vi "VM_Projeto.vi"() -> ()   [LabVIEW 2016]
uses:
  <vilib>/vision/Pattern Matching.llb/IMAQ Match Range Setting.ctl
  <vilib>/vision/Pattern Matching.llb/IMAQ Curve Parameters.ctl
  <vilib>/Analysis/_algsub.llb/Vector Norm Type.ctl
  <vilib>/Analysis/_algsub.llb/Real Vector Norm.vi
  <vilib>/vision/NI_Vision_Development_Module.lvlib
  <vilib>/Analysis/NI_AALPro.lvlib
panel:
  out "Array 5":i32[](array[numeric])
  out "reversed array":i32[](array[numeric])
  in  "stop":bool
  out "Array 4":T1[](array[typedef]) {"Contours"."Type" items=["No Selection", "Point", "Line", "Rectangle", "Oval", "Polygon", "Freehand Region", "Annulus", "Unused2", "Unused3", "Broken Line", "Freehand Line", "Rotated Rectangle"]}
  out "Array 3":cluster{"x":sgl, "y":sgl}[](array[cluster])
  out "Array 2":sgl[](array[numeric])
  out "Array":dbl[][](array[numeric])
  out "Number of Matches (filtered)":i32
  out "Number of Matches":i32
  in  "Number of Matches Requested":i32=40 min=1
  in  "Minimum Match Score":sgl=975.0 min=0 max=1000 format="%.2f"
  in  "Template":path=path "C:/Users/Alexandre/Documents/LabView Projects/Projeto/template.png"
  out "Image Out 2":T2(plugin-control)
  out "Image Out":T2(plugin-control)
  in  "Base":path=path "C:/Users/Alexandre/Documents/LabView Projects/Projeto/base.jpg"
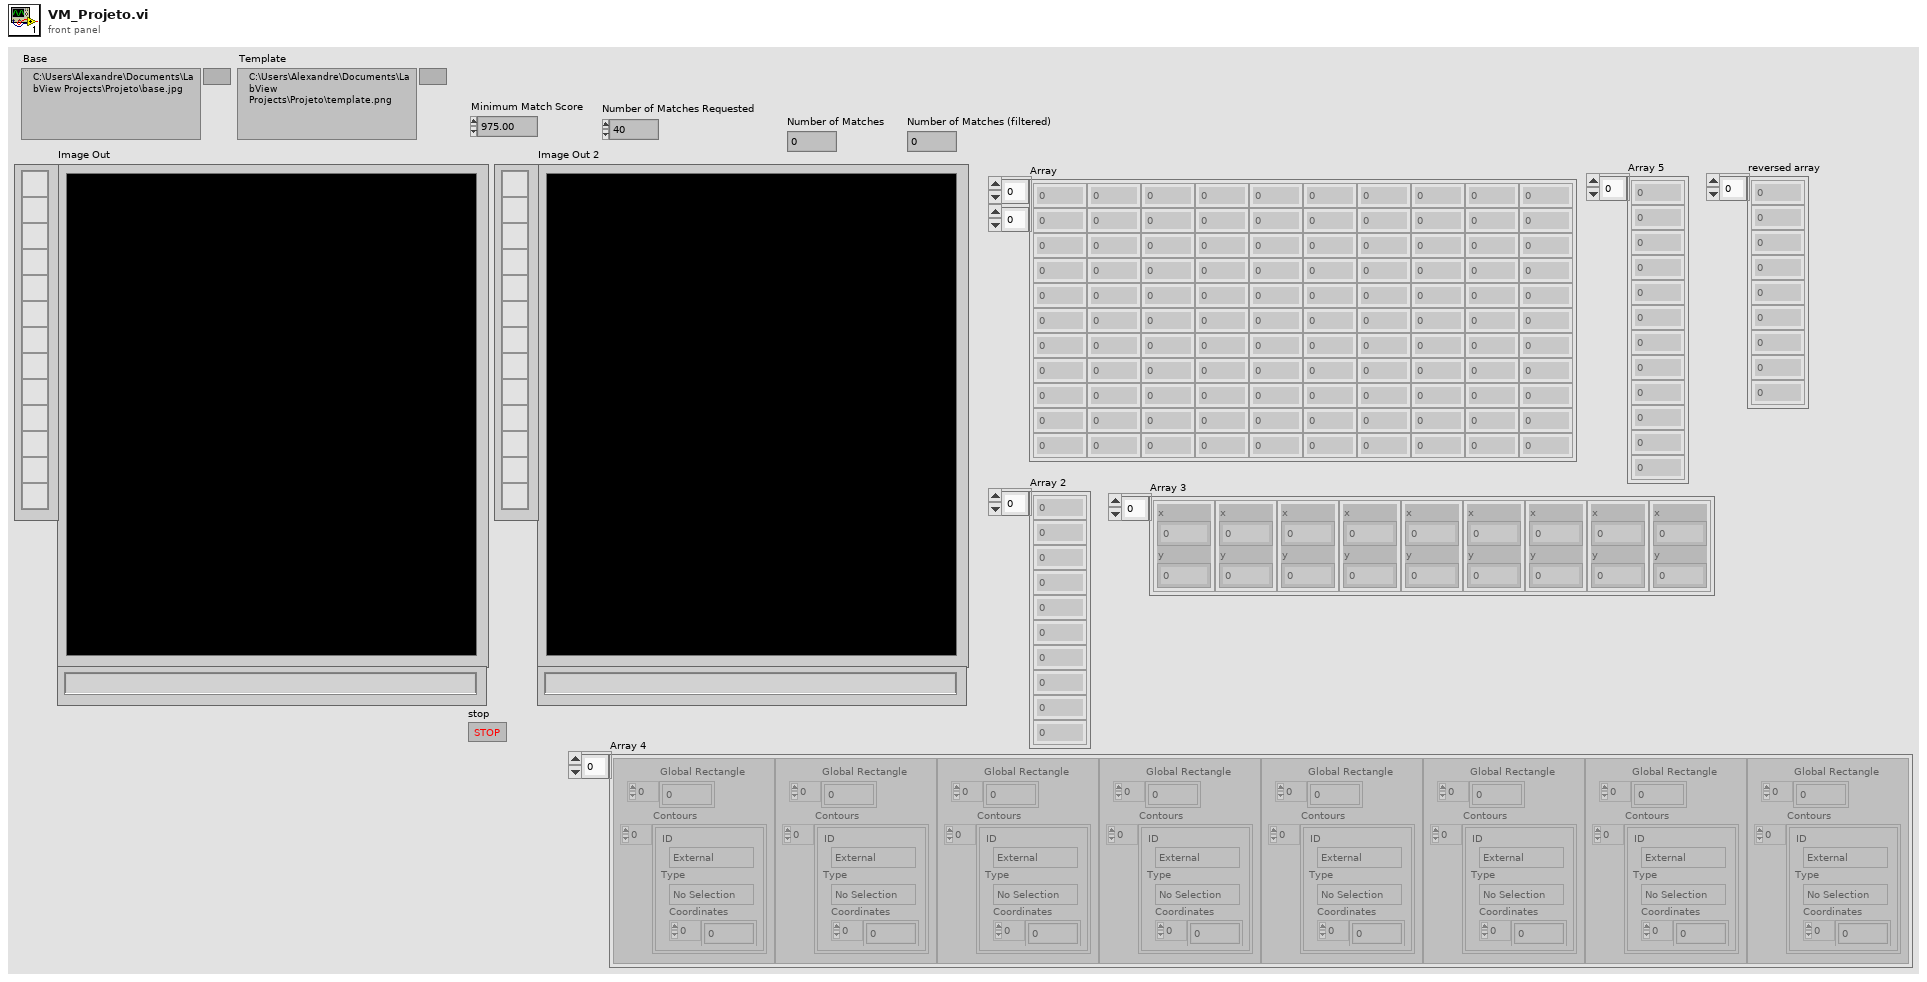
[diagram p1: front panel]
types:
  T1 = typedef "ROI Descriptor" = cluster{"Global Rectangle":i32[], "Contours":cluster{"ID":enum32{"External", "Internal"}, "Type":u32, "Coordinates":i32[]}[]}
  T2 = typedef "IMAQ Image.ctl" = refnum<image>
  T3 = typedef "IMAQ Curve Parameters.ctl" = cluster{"Extraction Mode":u32, "Edge Threshold":i32, "Edge Filter Size":u32, "Min Length":i32, "Row Search Step Size":i32, "Col Search Step Size":i32, "Max Endpoint Gap":i32, "Closed":bool, "Subpixel":bool}
  T4 = cluster{"Setup Data Item":u16, "Item Value":dbl}[]
  T5 = cluster{"Rotation":bool, "Scale":bool, "Occlusion":bool, "Reserved":bool, "Reserved":bool, "Reserved":bool}
  T6 = typedef "IMAQ Match Range Setting.ctl" = cluster{"Match Constraints":u32, "Min":dbl, "Max":dbl}
  T7 = typedef "IMAQ Rectangle" = cluster{"Left":i32, "Top":i32, "Right":i32, "Bottom":i32, "Rotation":dbl}
  T8 = typedef "Image Type" = u32
  T9 = typedef "IMAQ GM Match Report.ctl" = cluster{"Position":cluster{"x":sgl, "y":sgl}, "Angle":sgl, "Scale":sgl, "Score":sgl, "Bounding Box":cluster{"x":sgl, "y":sgl}[], "Contrast Reversed":bool, "Occlusion %":sgl, "Template Target Curve Score":sgl, "Target Template Curve Score":sgl, "Correlation Score":sgl}
  T10 = typedef "NI_AALPro.lvlib/Vector Norm Type.ctl" = u16
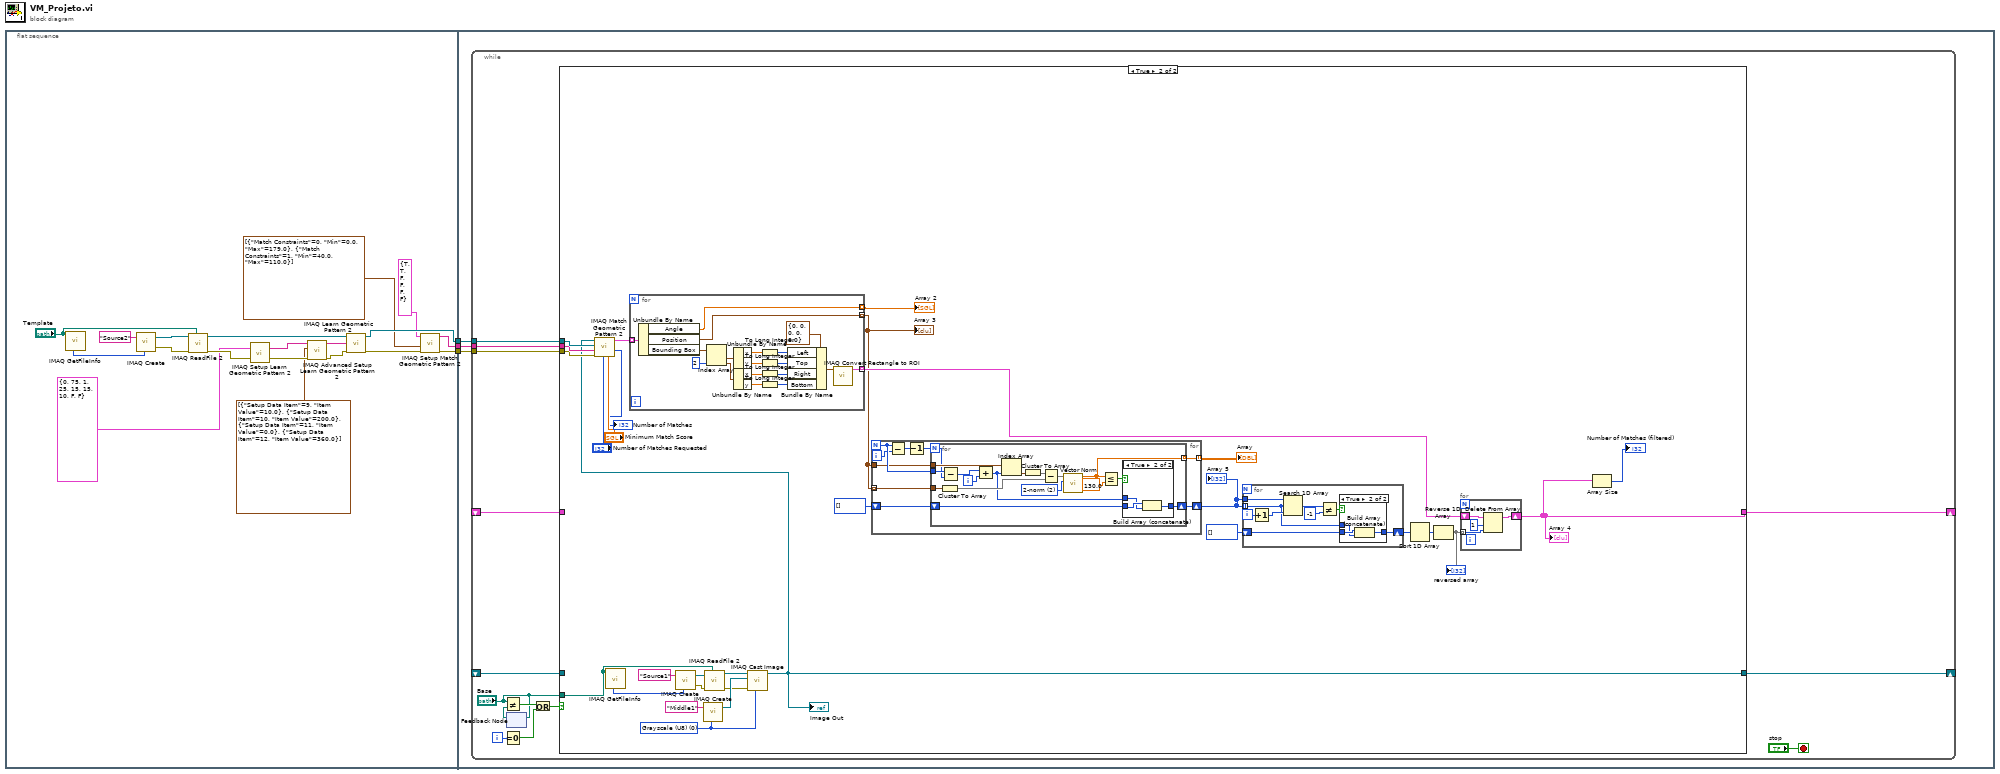
[diagram p0: block diagram]
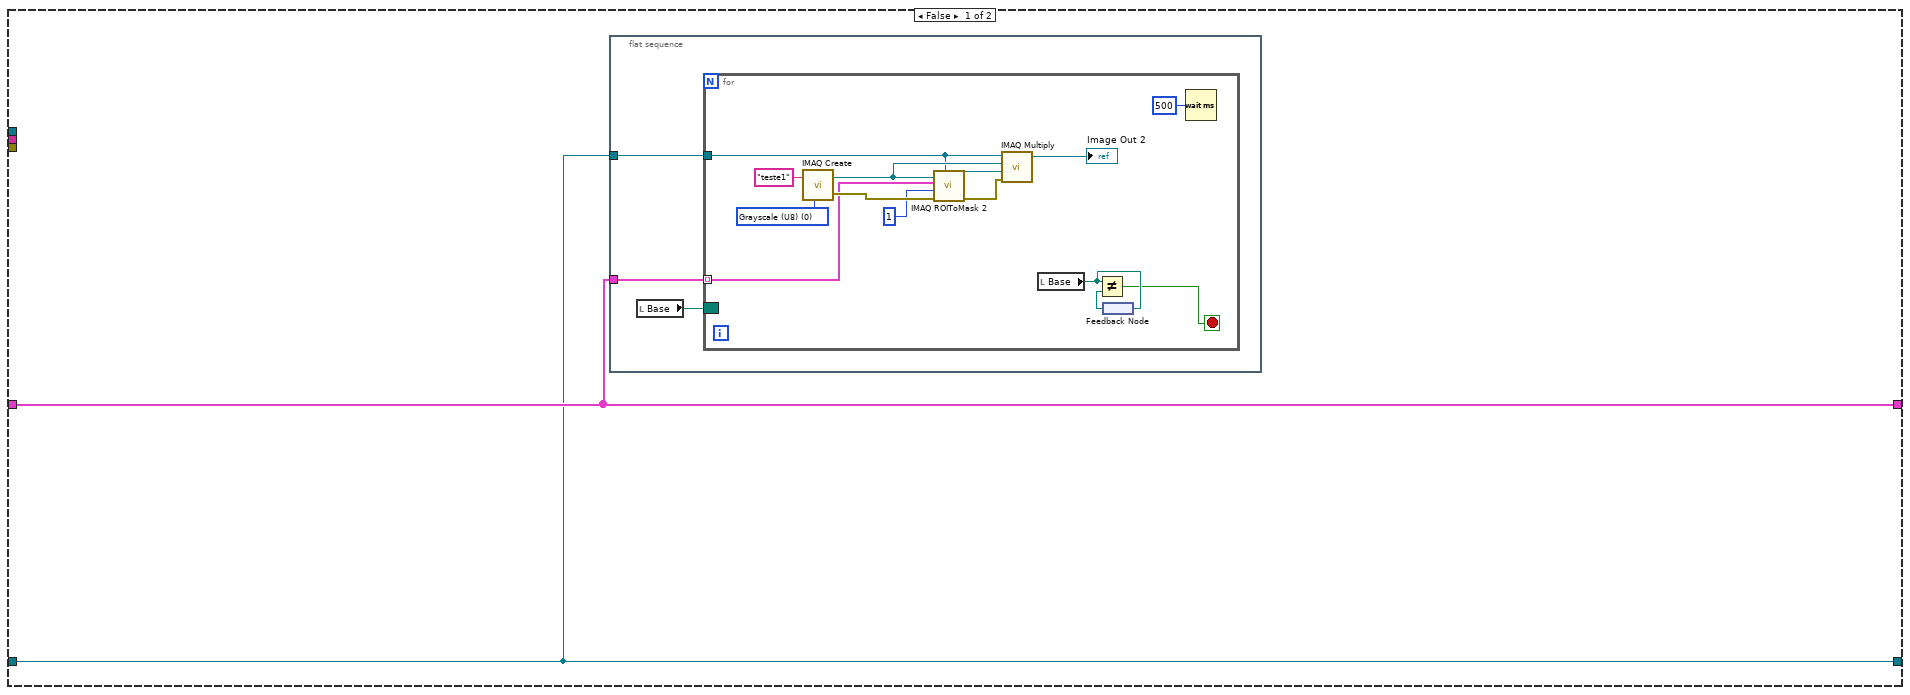
[diagram p2: hidden frame]
diagram:
  n1 = flat-sequence {
    tunnel: [w16] -> w3
    tunnel: [w14] -> w2
    tunnel: [w10] -> w1
    tunnel: w3 -> [w23]
    tunnel: w2 -> [w24]
    tunnel: w1 -> [w25]
    frame #0 {
      n2 = call "IMAQ GetFileInfo"("File Path"="Template") -> ("Image Type"=w18:T8)  [unwired: 4 in, 6 out]
      n3 = call "IMAQ Create"("Image Name"="Source2", "Image Type"=w18) -> ("New Image"=w21:T2, "error out"=w20:errorcluster)  [unwired: 3 in]
      n4 = call "IMAQ ReadFile 2"("File Path"="Template", "error in (no error)"=w20, "Image"=w21) -> ("error out"=w12:errorcluster, "Image Out"=w17:T2)  [unwired: 4 in, 3 out]
      n5 = call "IMAQ Setup Learn Geometric Pattern 2"("error in (no error)"=w12, "Curve Parameters"=T3 {"Extraction Mode"=0, "Edge Threshold"=75, "Edge Filter Size"=1, "Min Length"=25, "Row Search Step Size"=15, "Col Search Step Size"=15, "Max Endpoint Gap"=10, "Closed"=FALSE, "Subpixel"=FALSE}) -> ("error out"=w8:errorcluster, "Learn Geometric Pattern 2 Setup Data"=w9:string)
      n6 = call "IMAQ Advanced Setup Learn Geometric Pattern 2"("Learn Geometric Pattern 2 Setup Data In"=w9, "Advanced Geometric Learn Options 2"=T4 [{"Setup Data Item"=9, "Item Value"=10.0}, {"Setup Data Item"=10, "Item Value"=200.0}, {"Setup Data Item"=11, "Item Value"=0.0}, {"Setup Data Item"=12, "Item Value"=360.0}], "error in (no error)"=w8) -> ("Learn Geometric Pattern 2 Setup Data Out"=w7:string, "error out"=w6:errorcluster)  [unwired: 6 in]
      n7 = call "IMAQ Learn Geometric Pattern 2"("error in (no error)"=w6, "Learn Geometric Pattern 2 Setup Data"=w7, "Template Image"=w17) -> ("error out"=w11:errorcluster, "Template Image Out"=w16:T2)  [unwired: 7 in]
      n8 = call "IMAQ Setup Match Geometric Pattern 2"("error in (no error)"=w11, "Range Settings"=T6[] [{"Match Constraints"=0, "Min"=0.0, "Max"=179.0}, {"Match Constraints"=1, "Min"=40.0, "Max"=110.0}], "Match Mode"=T5 {"Rotation"=TRUE, "Scale"=TRUE, "Occlusion"=FALSE, "Reserved"=FALSE, "Reserved"=FALSE, "Reserved"=FALSE}) -> ("error out"=w10:errorcluster, "Match Geometric Pattern 2 Setup Data"=w14:string)  [unwired: 7 in]
    }
    frame #1 {
      n9 = while {
        shift-right: [w32] -> _
        shift-left: _ -> [w31]
        tunnel: w25 -> [w30]
        tunnel: w24 -> [w29]
        tunnel: w23 -> [w28]
        shift-right: [w27] -> _
        shift-left: _ -> [w26]
        i -> [w38]
        stop <- "stop" stop-if-true
        n10 = Equal To 0?(x=w38) -> (x = 0?=w36:bool)
        n11 = feedback-in #1("Base") -> ()
        n12 = feedback #1() -> (w37:path)  [unwired: 1 in]
        n13 = Not Equal?(x="Base", y=w37) -> (x != y?=w35:bool)
        n14 = Or(x=w35, y=w36) -> (x .or. y?=w34:bool)
        n15 = case shown="True" w34 {
          tunnel: "Base" -> [_ w79]
          tunnel: [w40 w62] -> w32
          tunnel: w31 -> [w40 _]
          tunnel: w30 -> [_ w63]
          tunnel: w29 -> [_ w64]
          tunnel: w28 -> [_ w65]
          tunnel: [w41 w66] -> w27
          tunnel: w26 -> [w41 _]
          frame False {
            n16 = flat-sequence {
              tunnel: w41 -> [w44]
              tunnel: w40 -> [w43]
              frame #0 {
                n17 = local read "Base"() -> (w42:path)
                n18 = for {
                  tunnel: w44 -> [w53] mode=indexing
                  tunnel: w43 -> [w50]
                  border: w42 -> [_]
                  stop <- w45 stop-if-true
                  w55 = T8 0 items=["Grayscale (U8)", "Grayscale (I16)", "Grayscale (SGL)", "Complex (CSG)", "RGB (U32)", "HSL (U32)", "RGB (U64)", "Grayscale (U16)"] ("Image Type")
                  n19 = call "IMAQ Create"("Image Name"="teste1", "Image Type"=w55) -> ("New Image"=w51:T2, "error out"=w58:errorcluster)  [unwired: 3 in]
                  n20 = call "IMAQ ROIToMask 2"("Image Model"=w50, "error in (no error)"=w58, "Filling Value (255)"=1, "ROI Descriptor"=w53, "Image"=w51) -> ("error out"=w52:errorcluster, "Image Out"=w56:T2)  [unwired: 4 in, 1 out]
                  n21 = call "IMAQ Multiply"("Image Src A"=w50, "Image Dst"=w51, "Image Src B"=w56, "error in (no error)"=w52) -> ("Image Dst Out"=→"Image Out 2":T2)  [unwired: 3 in, 1 out]
                  n22 = local read "Base"() -> (w46:path)
                  n23 = feedback-in #2(w46) -> ()
                  n24 = feedback #2() -> (w47:path)
                  n25 = Not Equal?(x=w46, y=w47) -> (x != y?=w45:bool)
                  n26 = Wait (ms)(milliseconds to wait=u32 500) -> ()  [unwired: 1 out]
                }
              }
            }
          }
          frame True {
            w88 = T8 0 items=["Grayscale (U8)", "Grayscale (I16)", "Grayscale (SGL)", "Complex (CSG)", "RGB (U32)", "HSL (U32)", "RGB (U64)", "Grayscale (U16)"] ("Image Type")
            n27 = call "IMAQ GetFileInfo"("File Path"=w79) -> ("Image Type"=w80:T8)  [unwired: 4 in, 6 out]
            n28 = call "IMAQ Create"("Image Name"="Source1", "Image Type"=w80) -> ("New Image"=w83:T2, "error out"=w82:errorcluster)  [unwired: 3 in]
            n29 = call "IMAQ Create"("Image Name"="Middle1", "Image Type"=w88) -> ("New Image"=w87:T2)  [unwired: 3 in, 1 out]
            n30 = call "IMAQ ReadFile 2"("File Path"=w79, "error in (no error)"=w82, "Image"=w83) -> ("error out"=w84:errorcluster, "Image Out"=w85:T2)  [unwired: 4 in, 3 out]
            n31 = call "IMAQ Cast Image"("Image Type"=w88, "error in (no error)"=w84, "Image Dst"=w87, "Image Src"=w85) -> ("Image Dst Out"=w62:T2)  [unwired: 6 in, 1 out]
            "Image Out" <- w62
            n32 = call "IMAQ Match Geometric Pattern 2"("Minimum Match Score"="Minimum Match Score", "Number of Matches Requested"="Number of Matches Requested", "error in (no error)"=w63, "Match Geometric Pattern 2 Setup Data"=w64, "Template Image"=w65, "Image"=w62) -> ("Number of Matches"=→"Number of Matches":i32, "Matches (pixel)"=w78:T9[])  [unwired: 2 in, 2 out]
            n33 = for {
              tunnel: w78 -> [w153] mode=indexing
              tunnel: [w138] -> w67 mode=indexing
              tunnel: [w137] -> w70 mode=indexing
              tunnel: [w136] -> w68 mode=indexing
              n34 = Unbundle By Name(w153) -> ("Angle"=w136:sgl, "Position"=w138:cluster{"x":sgl, "y":sgl}, "Bounding Box"=w151:cluster{"x":sgl, "y":sgl}[])
              n35 = Index Array(array=w151, index #2=2 ("index")) -> (element #1=w145:cluster{"x":sgl, "y":sgl}, element #2=w140:cluster{"x":sgl, "y":sgl})  [unwired: 1 in]
              n36 = Unbundle By Name(w145) -> ("x"=w144:sgl, "y"=w143:sgl)
              n37 = Unbundle By Name(w140) -> ("x"=w142:sgl, "y"=w141:sgl)
              n38 = To Long Integer(number=w144) -> (32bit integer=w149:i32)
              n39 = To Long Integer(number=w143) -> (32bit integer=w148:i32)
              n40 = To Long Integer(number=w142) -> (32bit integer=w147:i32)
              n41 = To Long Integer(number=w141) -> (32bit integer=w146:i32)
              n42 = Bundle By Name(cluster=T7 {"Left"=0, "Top"=0, "Right"=0, "Bottom"=0, "Rotation"=0.0} ("Rectangle"), "Left"=w149, "Top"=w148, "Right"=w147, "Bottom"=w146) -> (w139:T7)
              n43 = call "IMAQ Convert Rectangle to ROI"("Rectangle"=w139) -> ("ROI Descriptor"=w137:T1)  [unwired: 8 in, 1 out]
            }
            "Array 2" <- w68
            "Array 3" <- w67
            n44 = for {
              N -> [w114]
              tunnel: w67 -> [w113] mode=indexing
              tunnel: w67 -> [w112]
              shift-right: [w109] -> w73
              shift-left: i32[] [] -> [w111]
              tunnel: [w106] -> w76 mode=indexing
              i -> [w110]
              n45 = Subtract(x=w114, y=w110) -> (x-y=w108:i32)
              n46 = Decrement(x=w108) -> (x-1=w107:i32)
              n47 = for {
                N: w107 -> [w119]
                tunnel: w114 -> [w131]
                tunnel: w113 -> [w130]
                tunnel: w112 -> [w129]
                shift-right: [w120] -> w109
                shift-left: w111 -> [w121]
                tunnel: [w115] -> w106 mode=indexing
                i -> [w117]
                w124 = T10 2 items=["1-norm"=1, "2-norm"=2, "Inf-norm"=3, "-Inf-norm"=4, "User Defined"=5] ("norm type")
                n48 = Cluster To Array(cluster=w130) -> (array=w126:sgl[])
                n49 = Subtract(x=w131, y=w119) -> (x-y=w118:i32)
                n50 = Add(x=w118, y=w117) -> (x+y=w116:i32)
                n51 = Index Array(array=w129, index=w116) -> (element=w128:cluster{"x":sgl, "y":sgl})
                n52 = Cluster To Array(cluster=w128) -> (array=w127:sgl[])
                n53 = Subtract(x=w127, y=w126) -> (x-y=w125:sgl[])
                n54 = call-poly <vilib>:"Vector Norm.vi"("norm type"=w124, "Input Vector"=w125) -> ("norm"=w115:dbl)  [unwired: 8 in, 1 out]
                n55 = Less Or Equal?(x=w115, y=130.0) -> (x <= y?=w122:bool)
                n56 = case shown="True" w122 {
                  tunnel: w116 -> [_ w133]
                  tunnel: w121 -> [w132 w134]
                  tunnel: [w132 w135] -> w120
                  frame False {
                  }
                  frame True {
                    n57 = Build Array (concatenate)(w134, w133) -> (w135:i32[])
                  }
                }
              }
            }
            "Array" <- w76
            "Array 5" <- w73
            n58 = for {
              tunnel: w73 -> [w93] mode=indexing
              tunnel: w73 -> [w101]
              shift-right: [w95] -> w74
              shift-left: i32[] [] -> [w96]
              i -> [w94]
              n59 = Increment(x=w94) -> (x+1=w100:i32)
              n60 = Search 1D Array(1D array=w101, element=w93, start index (0)=w100) -> (index of element=w99:i32)
              n61 = Not Equal?(x=w99, y=-1) -> (x != y?=w97:bool)
              n62 = case shown="True" w97 {
                tunnel: w93 -> [_ w103]
                tunnel: w96 -> [w102 w105]
                tunnel: [w102 w104] -> w95
                frame False {
                }
                frame True {
                  n63 = Build Array (concatenate)(w105, w103) -> (w104:i32[])
                }
              }
            }
            n64 = Sort 1D Array(array=w74) -> (sorted array=w75:i32[])
            n65 = Reverse 1D Array(array=w75) -> (reversed array=w71:i32[])
            "reversed array" <- w71
            n66 = for {
              tunnel: w71 -> [w91] mode=indexing
              shift-right: [w89] -> w66
              shift-left: w70 -> [w92]
              n67 = Delete From Array(array=w92, length=1, index=w91) -> (array with subset deleted=w89:T1[])  [unwired: 1 out]
            }
            "Array 4" <- w66
            n68 = Array Size(array=w66) -> (size(s)=→"Number of Matches (filtered)":i32)
          }
        }
      }
    }
  }
